vi "Global-variables.vi"() -> ()   [LabVIEW 2015]
uses:
  <vilib>/userdefined/High Color/IMAQdx.ctl
panel:
  out "Exposure time rigth":dbl=10000.0
  out "Line rigth":dbl[](array[numeric])
  out "Line left":dbl[](array[numeric])
  out "Qualiy Map":bool
  out "Exposure time left":dbl=10000.0
  out "Stop":bool
  out "Camera-left":T1(plugin-control)
  in  "IMAQdx Session":T2
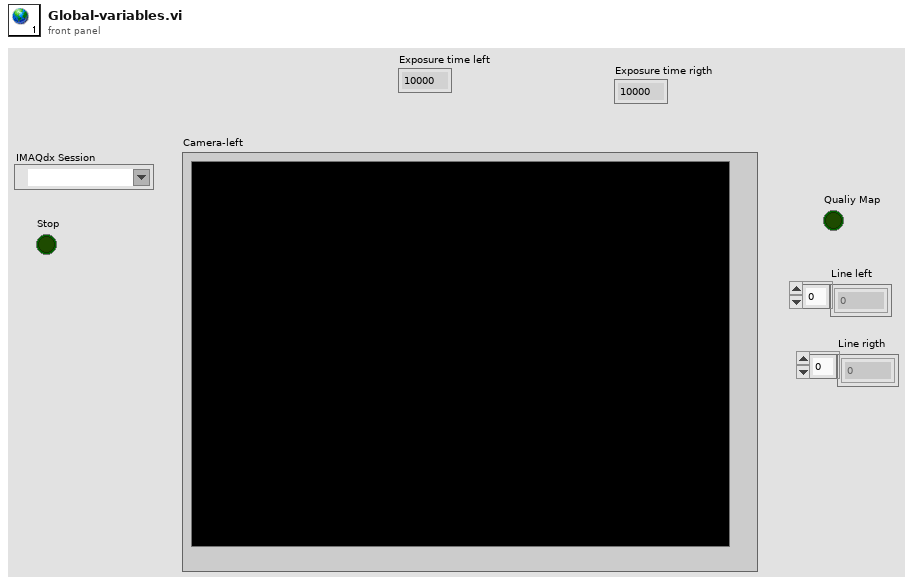
[diagram p1: front panel]
types:
  T1 = typedef "IMAQ Image.ctl" = refnum<image>
  T2 = typedef "IMAQdx.ctl" = refnum<k21>
diagram:
